vi "Difference Quotient.vi"   [LabVIEW 2016, in "xy_utilities.lvlib"]
doc: "Calculate the difference quotient (y[i-h/2]-y[i+h/s])/(x[i-h/2]-x[i+h/2]).\n\nWire data to the data input to determine the polymorphic instance to use or manually select the instance."
uses:
  xy_utilities.lvlib
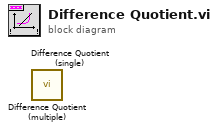
[diagram p0: block diagram]
diagram:
  n1 = call "Difference Quotient (multiple).vi"() -> ()  [unwired: 9 in, 3 out]
  n2 = call "Difference Quotient (single).vi"() -> ()  [unwired: 9 in, 3 out]
